vi "GetQueue.vi"(8 "error in (no error)":errorcluster, 10 "Sender":string, 11 "RemoteConnection In":refnum<class "RemoteConnection.lvclass">) -> (0 "error out":errorcluster, 2 "Queue":T1, 3 "RemoteConnection Out":refnum<class "RemoteConnection.lvclass">)   [LabVIEW 2013, in "RemoteConnection.lvclass"]
uses:
  RemoteConnection.lvclass
  message_queue.ctl
  Message/BaseMessage/BaseMessage.lvclass
  RemoteConnection.lvclass/RemoteConnection.ctl
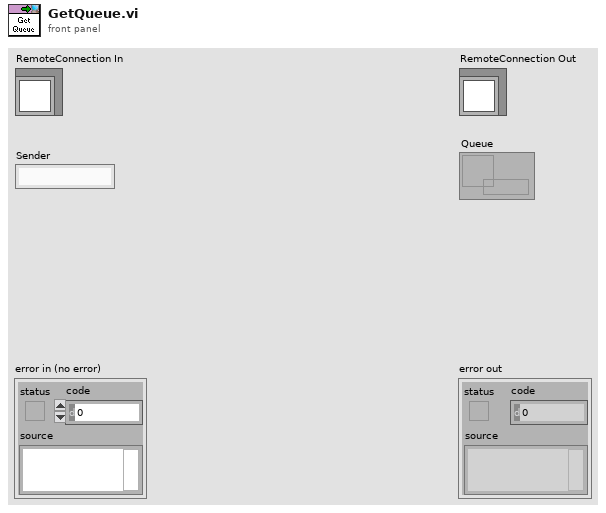
[diagram p1: front panel]
types:
  T1 = typedef "message_queue.ctl" = refnum<queue>
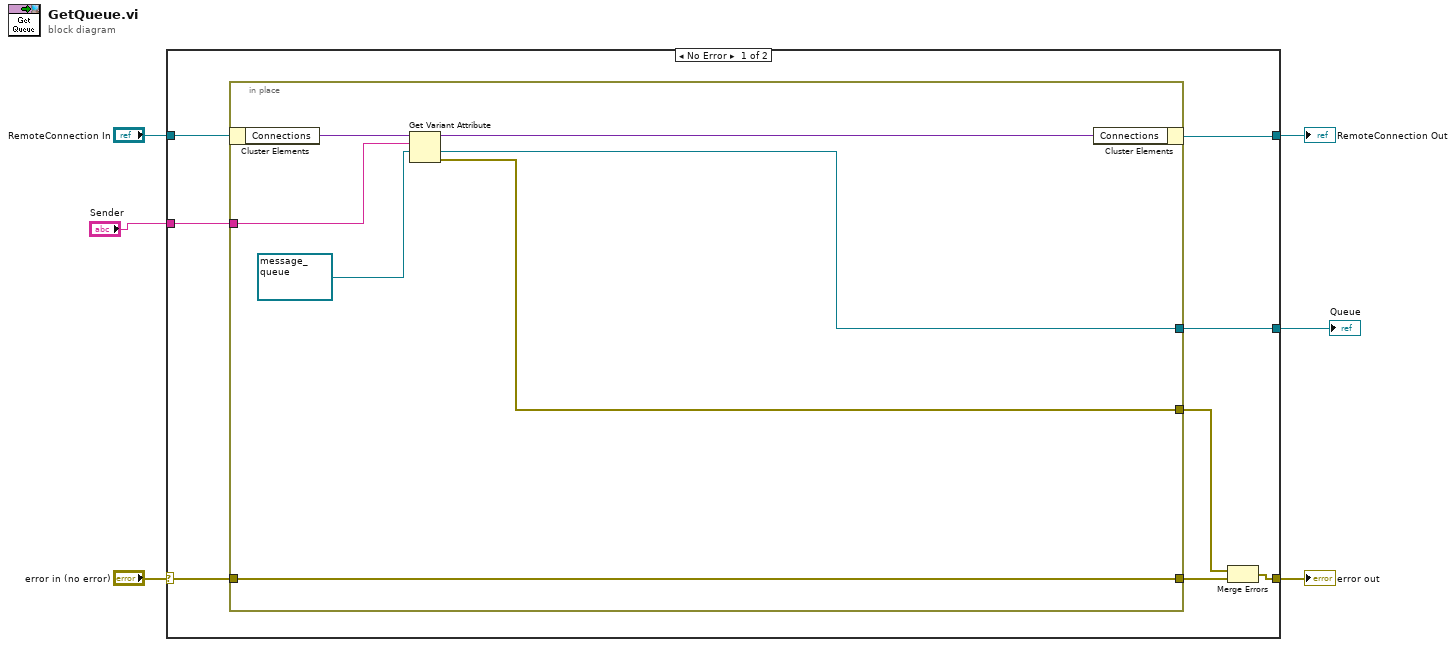
[diagram p0: block diagram]
diagram:
  n1 = case shown="No Error" "error in (no error)" {
    selector: "error in (no error)" -> [w12 w23]
    tunnel: [w9 w23] -> w4
    tunnel: [w13 w22] -> w5
    tunnel: "RemoteConnection In" -> [w14 w22]
    tunnel: "Sender" -> [w8 _]
    tunnel: [w7 _] -> w1
    frame No Error {
      n2 = in-place {
        in-place-border: w12 -> [w21]
        in-place-border: [w17] -> w11
        in-place-border: [w21] -> w10
        in-place-border: w8 -> [w19]
        in-place-border: [w15] -> w7
        n3 = in-place-cluster #1(w14) -> ("Connections"=w20:variant)
        n4 = Get Variant Attribute(Variant=w20, name=w19, default value (empty Variant)=T1 refnum ("Input queue")) -> (duplicate Variant=w18:variant, value=w15:T1, error out=w17:errorcluster)  [unwired: 1 in, 1 out]
        n5 = in-place-cluster #1("Connections"=w18) -> (w13:refnum<class "RemoteConnection.lvclass">)
      }
      n6 = Merge Errors(w11, w10) -> (w9:errorcluster)
    }
    frame Error {
    }
  }
  "error out" <- w4
  "RemoteConnection Out" <- w5
  "Queue" <- w1
